vi "selectcorrchan.vi"(0 "AO":bool) -> ()   [LabVIEW 2015]
panel:
  out "ne channel":string
  in  "Stop":bool
  in  "channels in":u16(ring) items=["Dev1/port0/line23", "Dev1/port0/line24", "Dev1/port0/line25", "Dev1/port0/line26", "Dev1/port0/line13"]
  # "Channel"
  # "does not exist: please choose corresponding\nexisting channel from list below"
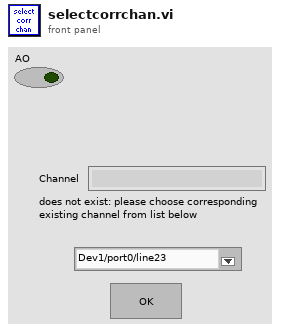
[diagram p1: front panel]
types:
  T1 = typedef "XYZStage.lvlib/XYZStage Configuration.ctl" = cluster{"VISA resource name":refnum<visa-resource-name>, "Timeout (3sec)":u32}
  T2 = cluster{"StageS":i32, "StageL":i32, "currmeas data dir":path, "image OD":u16, "contour OD":u16, "point OD":u16, "AOlines":tag[], "AIlines":tag[], "CI lines":tag[], "DO lines":tag[], "AO names":string[], "CI names":string[], "AI names":string[], "DO names":string[], "CIextensions":string[], "AIextensions":string[], "Voltage to Ygalvo":i32, "Voltage to Xgalvo":i32, "Voltage to patch":i32, "640 shutter":i32, "2P shutter":i32, "LT timestamp":u32, "Vp":i32, "Ip":i32, "camera trigger":i32, "master data dir":path, "voltage to Zpos":i32, "Vto2P":i32, "640 AO":i32, "488 AO":i32, "532 AO":i32, "640TTL":u32, "488TTL":u32, "532TTL":u32, "Device 1 sampleclock out":tag, "Device 1 Starttrigger out":tag, "Device 2 sampleclock in":tag, "Device 2 StartTrigger in ":tag, "2PODTTL":u32, "488 shutter":u32, "LCVR red":u32, "LCVR blue":u32, "Sutter Stage Config":T1}
  T3 = cluster{"newchan":cluster{"String":string, "value":i32}, "ne channel":string}
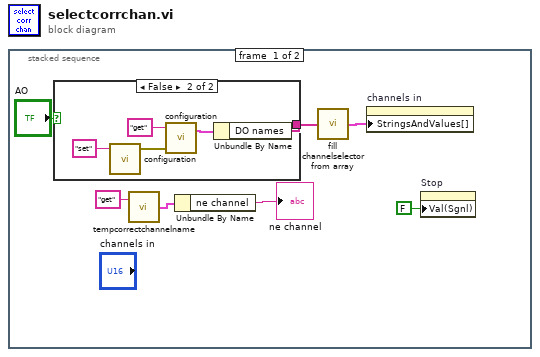
[diagram p0: block diagram]
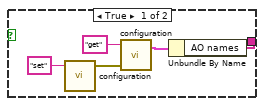
[diagram p2: hidden frame]
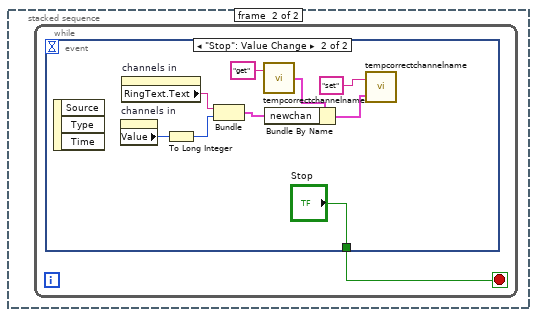
[diagram p3: hidden frame]
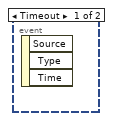
[diagram p4: hidden frame]
diagram:
  n1 = stacked-sequence {
    frame #0 {
      n2 = case shown="False" "AO" {
        tunnel: [w10 w15] -> w6
        frame True {
          n3 = call "configuration.vi"("command"="set") -> ("Error out"=w8:errorcluster)  [unwired: 2 in, 1 out]
          n4 = call "configuration.vi"("error in"=w8, "command"="get") -> ("config out"=w12:T2)  [unwired: 1 in, 1 out]
          n5 = Unbundle By Name(w12) -> ("AO names"=w10:string[])
        }
        frame False {
          n6 = call "configuration.vi"("command"="set") -> ("Error out"=w13:errorcluster)  [unwired: 2 in, 1 out]
          n7 = call "configuration.vi"("error in"=w13, "command"="get") -> ("config out"=w17:T2)  [unwired: 1 in, 1 out]
          n8 = Unbundle By Name(w17) -> ("DO names"=w15:string[])
        }
      }
      n9 = call "tempcorrectchannelname.vi"("command"="get") -> ("param out"=w3:T3)  [unwired: 1 in]
      n10 = Unbundle By Name(w3) -> ("ne channel"=→"ne channel":string)
      n11 = call "fill channelselector from array.vi"("channel  names"=w6) -> ("channel selector string and values"=w5:cluster{"String":string, "Value":u16}[])
      n12 = property on="channels in" class="Ring (strict)"("StringsAndValues[]"=w5) -> ()  [unwired: 2 in, 2 out]
      n13 = property on="Stop" class="Bool (strict)"("Val(Sgnl)"=FALSE ("Value (Signaling)")) -> ()  [unwired: 2 in, 2 out]
    }
    frame #1 {
      n14 = while {
        stop <- w18 stop-if-true
        n15 = event shown="[1] \"Stop\": Value Change" {
          selector: _ -> [_ _]
          dyn-events: _ -> [_ _]
          timeout: _ -> [_ _]
          tunnel: [_ "Stop"] -> w18
          event Timeout {
            n16 = event-data() -> ()  [unwired: 1 in, 3 out]
          }
          event "Stop": Value Change {
            n17 = event-data() -> ()  [unwired: 1 in, 3 out]
            n18 = property on="channels in" class="Ring (strict)"() -> ("Value"=w25:u16)  [unwired: 2 in, 2 out]
            n19 = property on="channels in" class="Ring (strict)"() -> ("RingText.Text"=w26:string)  [unwired: 2 in, 2 out]
            n20 = To Long Integer(number=w25) -> (32bit integer=w19:i32)
            n21 = Bundle("RingText.Text"=w26, w19) -> (w21:cluster{"RingText.Text":string, i32})  [unwired: 1 in]
            n22 = call "tempcorrectchannelname.vi"("command"="get") -> ("param out"=w22:T3)  [unwired: 1 in]
            n23 = Bundle By Name(cluster=w22, "newchan"=w21) -> (w20:T3)
            n24 = call "tempcorrectchannelname.vi"("param in"=w20, "command"="set") -> ()  [unwired: 1 out]
          }
        }
      }
    }
  }
